vi "CRYCalc Ppk value.vi"(0 "Data values in":T1 {"Z data" items=["dB", "Lin"]; "X data" items=["dB", "Lin"]; "Y data" items=["dB", "Lin"]; "Z dB ref" format="%.1f"; "Z axis" items=["Log", "Lin"]; "X dB ref" format="%.1f"; "X axis" items=["Log", "Lin"]; "Y axis" items=["Log", "Lin"]; "Y dB ref" format="%.1f"; "Curve"."z" format="%.2f"; "Curve"."y" format="%.2f"; "Curve"."x" format="%.2f"}, 1 "Step Setup VI No":i32, 5 "USL":dbl, 7 "LSL":dbl, 11 "Statistic Run Number":i32, 12 "Work in":u16, 13 "Mode xyz":u16) -> (4 "Ppk value Out":T1 {"Z data" items=["dB", "Lin"]; "X data" items=["dB", "Lin"]; "Y data" items=["dB", "Lin"]; "Z dB ref" format="%.1f"; "Z axis" items=["Log", "Lin"]; "X dB ref" format="%.1f"; "X axis" items=["Log", "Lin"]; "Y axis" items=["Log", "Lin"]; "Y dB ref" format="%.1f"; "Curve"."z" format="%.2f"; "Curve"."y" format="%.2f"; "Curve"."x" format="%.2f"}, 6 "Mean Out":T1 {"Z data" items=["dB", "Lin"]; "X data" items=["dB", "Lin"]; "Y data" items=["dB", "Lin"]; "Z dB ref" format="%.1f"; "Z axis" items=["Log", "Lin"]; "X dB ref" format="%.1f"; "X axis" items=["Log", "Lin"]; "Y axis" items=["Log", "Lin"]; "Y dB ref" format="%.1f"; "Curve"."z" format="%.2f"; "Curve"."y" format="%.2f"; "Curve"."x" format="%.2f"}, 10 "Absolute StanDev Out":T1 {"Z data" items=["dB", "Lin"]; "X data" items=["dB", "Lin"]; "Y data" items=["dB", "Lin"]; "Z dB ref" format="%.1f"; "Z axis" items=["Log", "Lin"]; "X dB ref" format="%.1f"; "X axis" items=["Log", "Lin"]; "Y axis" items=["Log", "Lin"]; "Y dB ref" format="%.1f"; "Curve"."z" format="%.2f"; "Curve"."y" format="%.2f"; "Curve"."x" format="%.2f"})   [LabVIEW 2013]
uses:
  Typedef Control/CRYData Cluster Array.ctl
  Typedef Control/CRYData Cluster.ctl
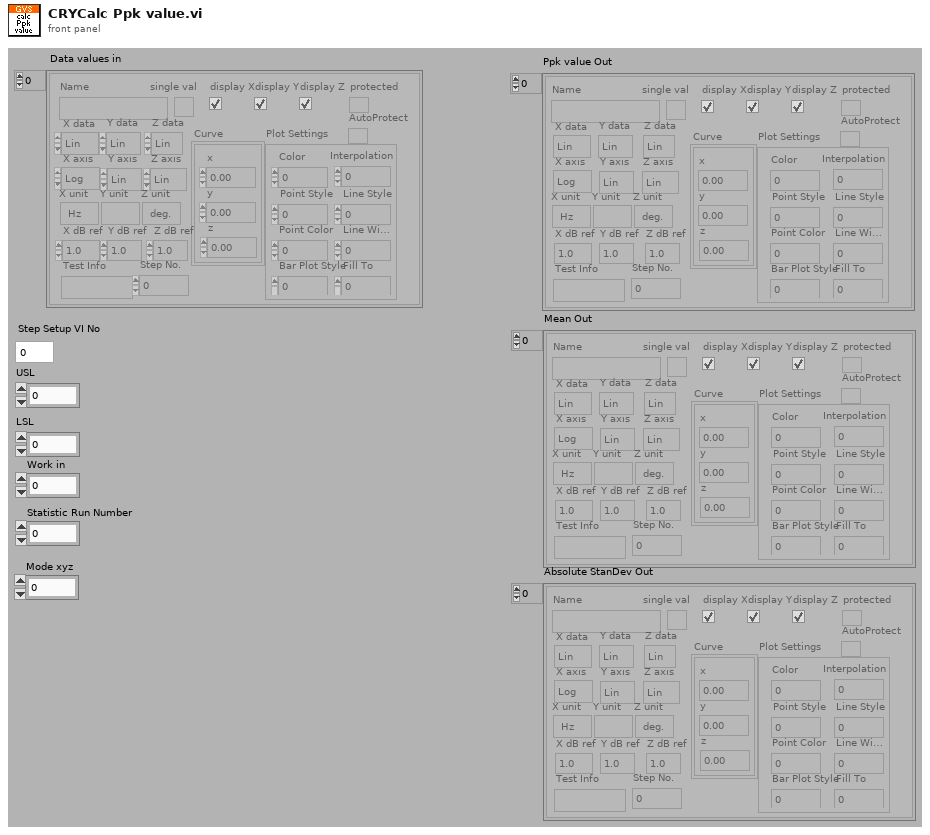
[diagram p1: front panel]
types:
  T1 = typedef "CRYData Cluster Array.ctl" = T2[]
  T2 = typedef "CRYData Cluster.ctl" = cluster{"Name":string, "Curve":cluster{"x":dbl, "y":dbl, "z":dbl}[], "X data":u16, "Y data":u16, "Z data":u16, "X axis":u16, "Y axis":u16, "Z axis":u16, "X unit":string, "Y unit":string, "Z unit":string, "X dB ref":dbl, "Y dB ref":dbl, "Z dB ref":dbl, "single val":bool, "protected":bool, "display X":bool, "display Y":bool, "display Z":bool, "Test Info":string, "Step No.":i32, "Plot Settings":cluster{"Color":u32, "Interpolation":u8, "Point Style":u8, "Line Style":u8, "Point Color":u32, "Line Width":u8, "Bar Plot Style":u8, "Fill To":i16}, "AutoProtect":bool}
  T3 = enum32{"English", "Chinese", "Korean", "Japanese", "Russian", "Chinese traditional"}
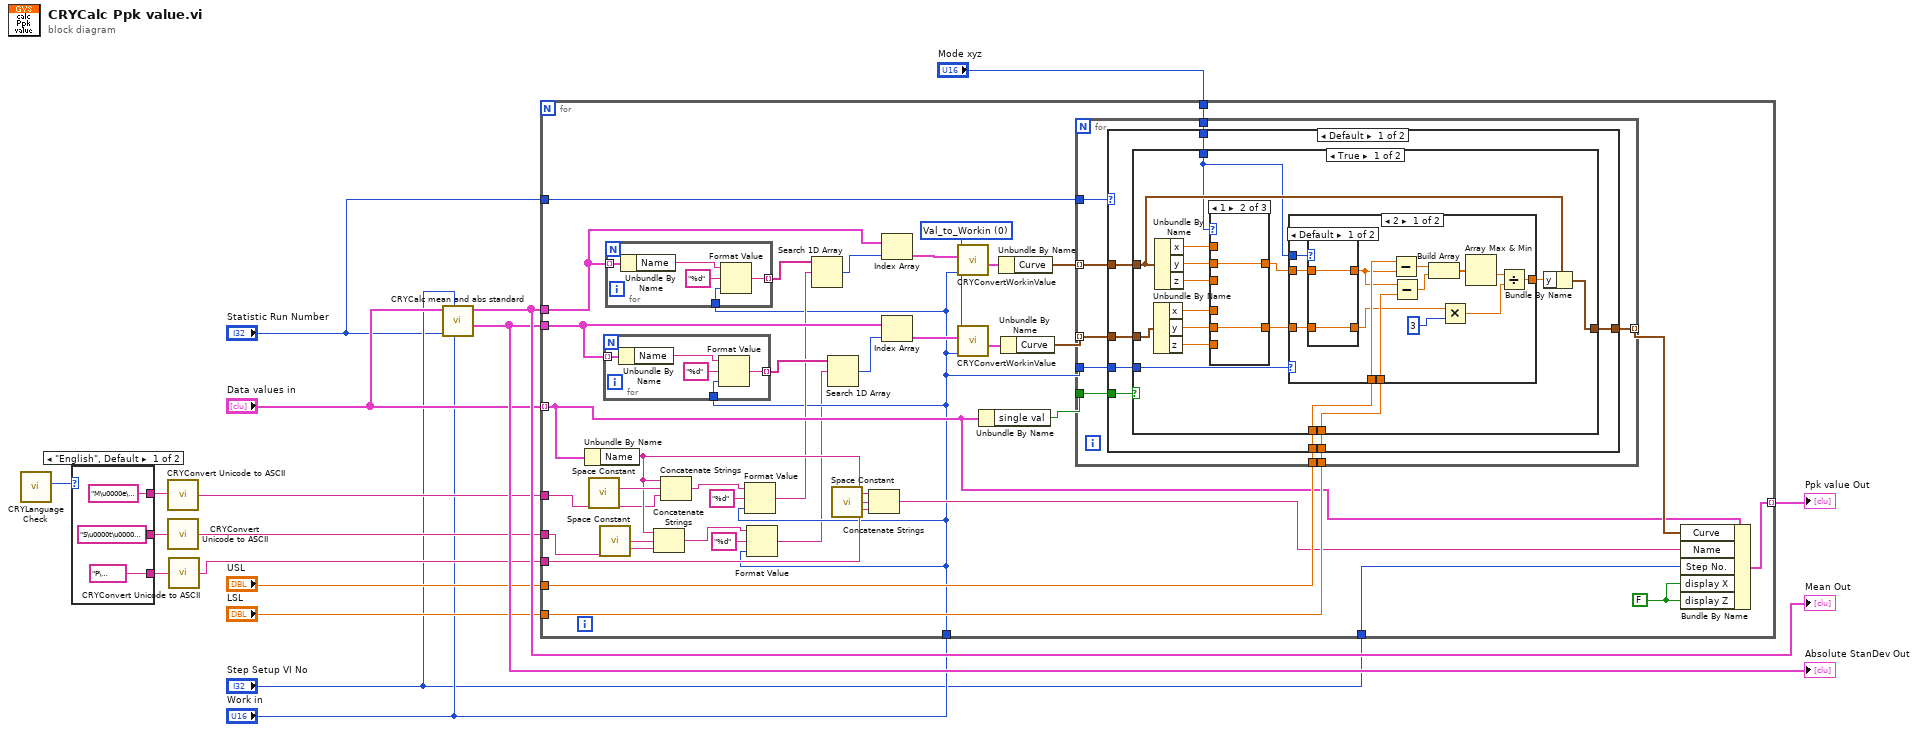
[diagram p0: block diagram]
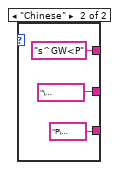
[diagram p2: hidden frame]
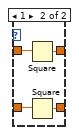
[diagram p5: hidden frame]
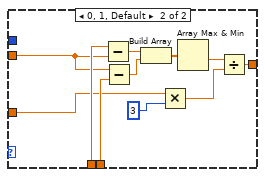
[diagram p6: hidden frame]
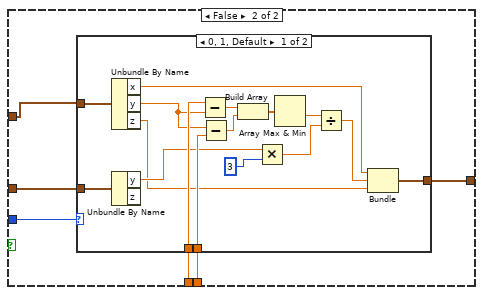
[diagram p7: hidden frame]
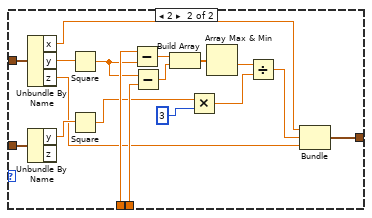
[diagram p8: hidden frame]
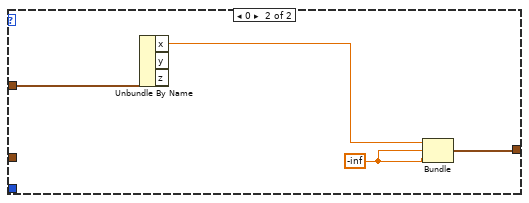
[diagram p9: hidden frame]
diagram:
  n1 = call "CRYLanguage Check.vi"() -> ("Language"=w10:T3)  [unwired: 10 in, 1 out]
  n2 = case shown="\"English\", Default" w10 {
    tunnel: ["M\u0000e\u0000a\u0000n\u0000" ("format string") "s^GW<P" ("format string")] -> w11
    tunnel: ["S\u0000t\u0000d\u0000 \u0000D\u0000e\u0000v\u0000" ("format string") "\u0007hÆQî]" ("format string")] -> w9
    tunnel: ["P\u0000p\u0000k\u0000" "P\u0000p\u0000k\u0000" ("format string")] -> w8
    frame "English", Default {
    }
    frame "Chinese" {
    }
  }
  n3 = call "CRYConvert Unicode to ASCII.vi"("Unicode"=w11) -> ("ASCII"=w7:string)  [unwired: 4 in]
  n4 = call "CRYConvert Unicode to ASCII.vi"("Unicode"=w9) -> ("ASCII"=w6:string)  [unwired: 4 in]
  n5 = call "CRYConvert Unicode to ASCII.vi"("Unicode"=w8) -> ("ASCII"=w5:string)  [unwired: 4 in]
  n6 = call "CRYCalc mean and abs standard.vi"("Work in"="Work in", "Step Setup VI No"="Step Setup VI No", "Statistic Run Number"="Statistic Run Number", "Data in"="Data values in") -> ("Absolute StanDev Out"=w16:T1, "Mean Out"=w17:T1)  [unwired: 5 in, 1 out]
  "Mean Out" <- w17
  "Absolute StanDev Out" <- w16
  n7 = for {
    tunnel: w17 -> [w34]
    tunnel: w16 -> [w32]
    tunnel: "Data values in" -> [w38] mode=indexing
    tunnel: "USL" -> [w57]
    tunnel: "LSL" -> [w56]
    tunnel: [w40] -> w12 mode=indexing
    tunnel: "Step Setup VI No" -> [w49]
    tunnel: w7 -> [w48]
    tunnel: w6 -> [w47]
    tunnel: w5 -> [w46]
    tunnel: "Work in" -> [w25]
    tunnel: "Statistic Run Number" -> [w39]
    tunnel: "Mode xyz" -> [w36]
    w35 = FALSE ("display Z")
    w41 = u16 0 items=["Val_to_Workin", "Workin_to_ Val"] ("Type")
    n8 = Unbundle By Name(w38) -> ("Name"=w53:string)
    n9 = call <vilib>:"Space Constant.vi"() -> ("String"=w61:string)
    n10 = call <vilib>:"Space Constant.vi"() -> ("String"=w60:string)
    n11 = for {
      tunnel: w32 -> [w66] mode=indexing
      tunnel: w25 -> [w63]
      tunnel: [w62] -> w31 mode=indexing
      n12 = Unbundle By Name(w66) -> ("Name"=w64:string)
      n13 = Format Value(string ("")=w64, format string="%d", value (0)=w63) -> (output string=w62:string)
    }
    n14 = for {
      tunnel: w34 -> [w71] mode=indexing
      tunnel: w25 -> [w68]
      tunnel: [w67] -> w33 mode=indexing
      n15 = Unbundle By Name(w71) -> ("Name"=w69:string)
      n16 = Format Value(string ("")=w69, format string="%d", value (0)=w68) -> (output string=w67:string)
    }
    n17 = Concatenate Strings(w53, w60, w47) -> (w26:string)
    n18 = Concatenate Strings(w53, w61, w48) -> (w29:string)
    n19 = Format Value(string ("")=w29, format string="%d", value (0)=w25) -> (output string=w27:string)
    n20 = Format Value(string ("")=w26, format string="%d", value (0)=w25) -> (output string=w24:string)
    n21 = Search 1D Array(1D array=w33, element=w27) -> (index of element=w59:i32)  [unwired: 1 in]
    n22 = Search 1D Array(1D array=w31, element=w24) -> (index of element=w58:i32)  [unwired: 1 in]
    n23 = call <vilib>:"Space Constant.vi"() -> ("String"=w54:string)
    n24 = Concatenate Strings(w53, w54, w46) -> (w52:string)
    n25 = Index Array(array=w34, index=w59) -> (element=w45:T2)
    n26 = Index Array(array=w32, index=w58) -> (element=w43:T2)
    n27 = call "CRYConvertWorkinValue.vi"("Work in"=w25, "In"=w45, "Type"=w41) -> ("Out"=w44:T2)  [unwired: 8 in]
    n28 = call "CRYConvertWorkinValue.vi"("Work in"=w25, "In"=w43, "Type"=w41) -> ("Out"=w42:T2)  [unwired: 8 in]
    n29 = Unbundle By Name(w38) -> ("single val"=w37:bool)
    n30 = Unbundle By Name(w44) -> ("Curve"=w51:cluster{"x":dbl, "y":dbl, "z":dbl}[])
    n31 = Unbundle By Name(w42) -> ("Curve"=w50:cluster{"x":dbl, "y":dbl, "z":dbl}[])
    n32 = for {
      tunnel: w57 -> [w80]
      tunnel: w56 -> [w79]
      tunnel: [w78] -> w55 mode=indexing
      tunnel: w51 -> [w77] mode=indexing
      tunnel: w50 -> [w76] mode=indexing
      tunnel: w25 -> [w75]
      tunnel: w39 -> [w74]
      tunnel: w37 -> [w73]
      tunnel: w36 -> [w72]
      n33 = case shown="Default" w74 {
        tunnel: w80 -> [w88 _]
        tunnel: w79 -> [w87 _]
        tunnel: [w86 w185] -> w78
        tunnel: w77 -> [w85 w184]
        tunnel: w76 -> [w84 _]
        tunnel: w75 -> [w83 _]
        tunnel: w73 -> [w82 _]
        tunnel: w72 -> [w81 _]
        frame Default {
          n34 = case shown="True" w82 {
            tunnel: w88 -> [w104 w147]
            tunnel: w87 -> [w103 w146]
            tunnel: [w90 w145] -> w86
            tunnel: w85 -> [w91 w144]
            tunnel: w84 -> [w102 w143]
            tunnel: w83 -> [w101 w142]
            tunnel: w81 -> [w89 _]
            frame True {
              n35 = Unbundle By Name(w102) -> ("x"=w97:dbl, "y"=w96:dbl, "z"=w95:dbl)
              n36 = Unbundle By Name(w91) -> ("x"=w100:dbl, "y"=w99:dbl, "z"=w98:dbl)
              n37 = case shown="1" w89 {
                tunnel: w100 -> [w106 _ _]
                tunnel: w99 -> [_ w108 _]
                tunnel: w98 -> [_ _ w110]
                tunnel: w97 -> [w105 _ _]
                tunnel: w96 -> [_ w107 _]
                tunnel: w95 -> [_ _ w109]
                tunnel: [w106 w108 w110] -> w94
                tunnel: [w105 w107 w109] -> w93
                frame 0, Default {
                }
                frame 1 {
                }
                frame 2 {
                }
              }
              n38 = case shown="2" w101 {
                tunnel: w104 -> [w118 w135]
                tunnel: w103 -> [w117 w134]
                tunnel: w94 -> [w114 w132]
                tunnel: w93 -> [w113 w131]
                tunnel: [w112 w133] -> w92
                tunnel: w89 -> [w111 _]
                frame 2 {
                  n39 = case shown="Default" w111 {
                    tunnel: [w126 w130] -> w116
                    tunnel: [w125 w129] -> w115
                    tunnel: w114 -> [w126 w128]
                    tunnel: w113 -> [w125 w127]
                    frame Default {
                    }
                    frame 1 {
                      n40 = Square(x=w128) -> (x^2=w130:dbl)
                      n41 = Square(x=w127) -> (x^2=w129:dbl)
                    }
                  }
                  n42 = Subtract(x=w118, y=w116) -> (x-y=w119:dbl)
                  n43 = Subtract(x=w116, y=w117) -> (x-y=w120:dbl)
                  n44 = Build Array(w119, w120) -> (w121:dbl[])
                  n45 = Multiply(x=w115, y=3 ("standard deviation")) -> (x*y=w124:dbl)
                  n46 = Array Max & Min(array=w121) -> (min value=w123:dbl)  [unwired: 3 out]
                  n47 = Divide(x=w123, y=w124) -> (x/y=w112:dbl)
                }
                frame 0, 1, Default {
                  n48 = Subtract(x=w135, y=w132) -> (x-y=w136:dbl)
                  n49 = Subtract(x=w132, y=w134) -> (x-y=w137:dbl)
                  n50 = Build Array(w136, w137) -> (w138:dbl[])
                  n51 = Multiply(x=w131, y=3 ("standard deviation")) -> (x*y=w141:dbl)
                  n52 = Array Max & Min(array=w138) -> (min value=w140:dbl)  [unwired: 3 out]
                  n53 = Divide(x=w140, y=w141) -> (x/y=w133:dbl)
                }
              }
              n54 = Bundle By Name(cluster=w91, "y"=w92) -> (w90:cluster{"x":dbl, "y":dbl, "z":dbl})
            }
            frame False {
              n55 = case shown="0, 1, Default" w142 {
                tunnel: w147 -> [w155 w173]
                tunnel: w146 -> [w154 w172]
                tunnel: [w153 w164] -> w145
                tunnel: w144 -> [w152 w169]
                tunnel: w143 -> [w151 w168]
                frame 0, 1, Default {
                  n56 = Unbundle By Name(w152) -> ("x"=w156:dbl, "y"=w150:dbl, "z"=w148:dbl)
                  n57 = Unbundle By Name(w151) -> ("y"=w149:dbl)  [unwired: 1 out]
                  n58 = Subtract(x=w155, y=w150) -> (x-y=w157:dbl)
                  n59 = Subtract(x=w150, y=w154) -> (x-y=w158:dbl)
                  n60 = Build Array(w157, w158) -> (w159:dbl[])
                  n61 = Multiply(x=w149, y=3 ("standard deviation")) -> (x*y=w162:dbl)
                  n62 = Array Max & Min(array=w159) -> (min value=w161:dbl)  [unwired: 3 out]
                  n63 = Divide(x=w161, y=w162) -> (x/y=w163:dbl)
                  n64 = Bundle("x"=w156, w163, "z"=w148) -> (w153:cluster{"x":dbl, dbl, "z":dbl})  [unwired: 1 out]
                }
                frame 2 {
                  n65 = Unbundle By Name(w169) -> ("x"=w174:dbl, "y"=w171:dbl, "z"=w165:dbl)
                  n66 = Unbundle By Name(w168) -> ("y"=w170:dbl)  [unwired: 1 out]
                  n67 = Square(x=w171) -> (x^2=w167:dbl)
                  n68 = Square(x=w170) -> (x^2=w166:dbl)
                  n69 = Subtract(x=w173, y=w167) -> (x-y=w175:dbl)
                  n70 = Subtract(x=w167, y=w172) -> (x-y=w176:dbl)
                  n71 = Build Array(w175, w176) -> (w177:dbl[])
                  n72 = Multiply(x=w166, y=3 ("standard deviation")) -> (x*y=w180:dbl)
                  n73 = Array Max & Min(array=w177) -> (min value=w179:dbl)  [unwired: 3 out]
                  n74 = Divide(x=w179, y=w180) -> (x/y=w181:dbl)
                  n75 = Bundle("x"=w174, w181, "z"=w165) -> (w164:cluster{"x":dbl, dbl, "z":dbl})  [unwired: 1 out]
                }
              }
            }
          }
        }
        frame 0 {
          w182 = -inf
          n76 = Unbundle By Name(w184) -> ("x"=w183:dbl)  [unwired: 2 out]
          n77 = Bundle("x"=w183, w182, w182) -> (w185:cluster{"x":dbl, dbl, dbl})  [unwired: 1 out]
        }
      }
    }
    n78 = Bundle By Name(cluster=w38, "Curve"=w55, "Name"=w52, "Step No."=w49, "display X"=w35, "display Z"=w35) -> (w40:T2)
  }
  "Ppk value Out" <- w12
